vi "Evaluate Part 1.vi"() -> ()   [LabVIEW 2021]
uses:
  Proto/Module.lvclass
panel:
  out "Low Pulses":i32
  out "High Pulses":i32
  out "delimited string":string
  out "High x Low":u64
  in  "Input":string
  # "2532512431 too high"
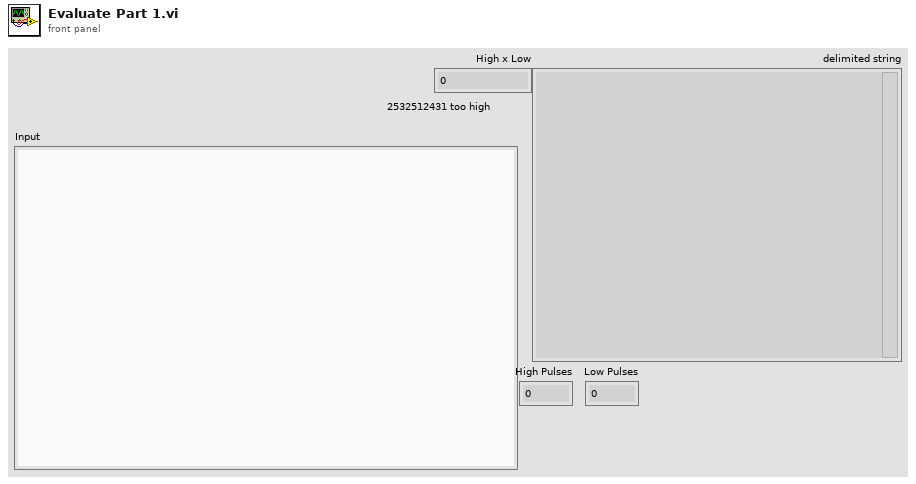
[diagram p1: front panel]
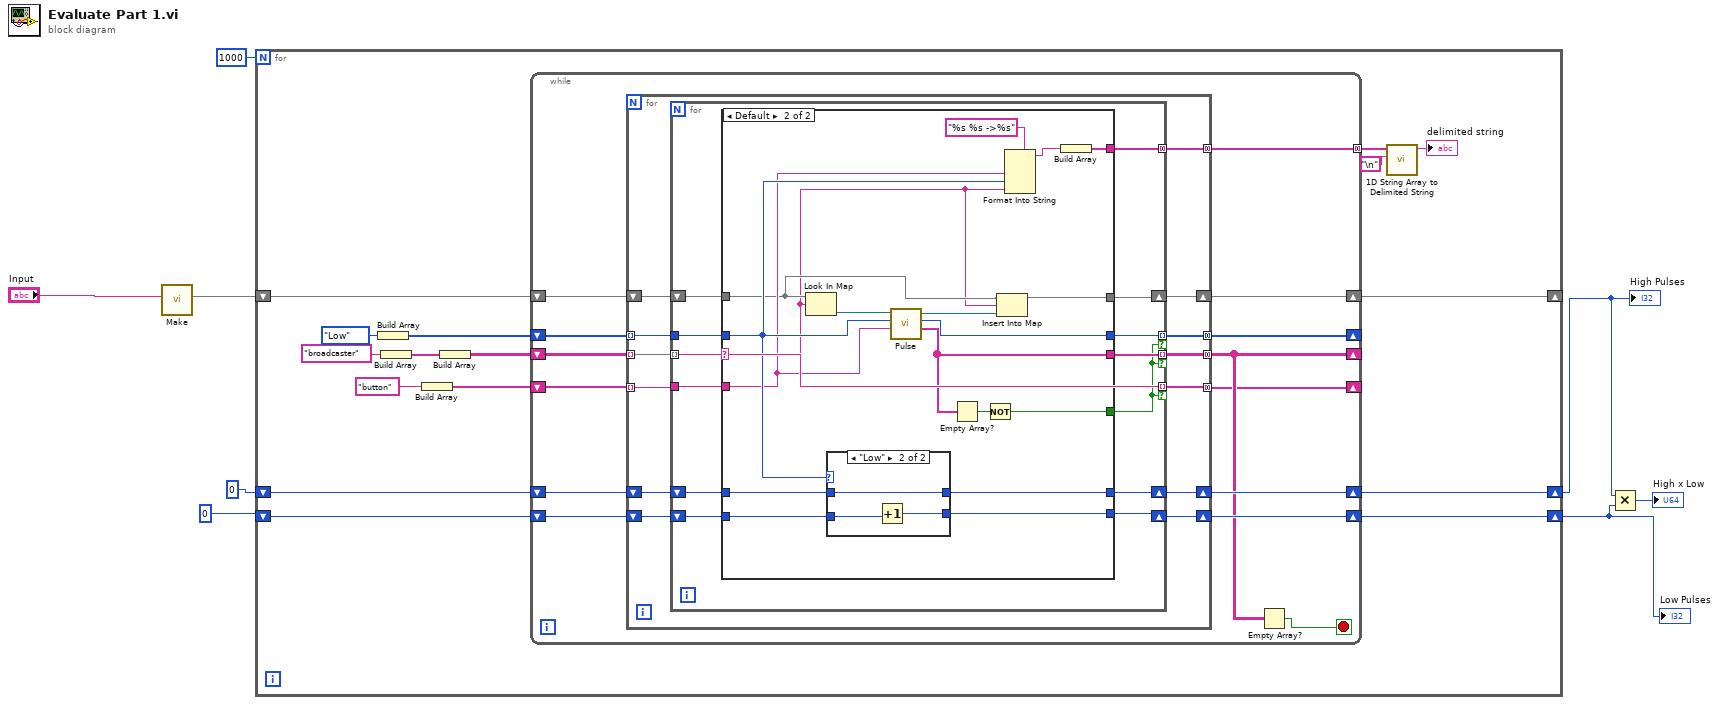
[diagram p0: block diagram]
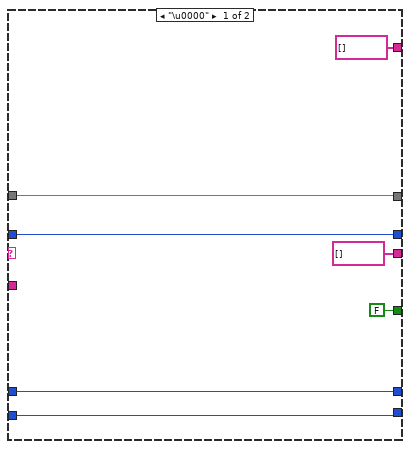
[diagram p2: hidden frame]
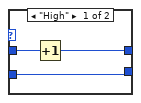
[diagram p3: hidden frame]
diagram:
  n1 = call "Make.vi"("Input"="Input") -> ("map"=w8:map{string, refnum<class "Module.lvclass">})  [unwired: 8 in, 2 out]
  n2 = for {
    N: 1000 -> [_]
    shift-right: [w11] -> _
    shift-left: w8 -> [w24]
    shift-right: [w18] -> w6
    shift-left: u64 0 -> [w10]
    shift-right: [w12] -> w4
    shift-left: u64 0 -> [w9]
    n3 = Build Array(enum16{"Low", "High"}."Low" ("Pulse In")) -> (w19:enum16{"Low", "High"}[])
    n4 = Build Array("broadcaster" ("key")) -> (w21:string[])
    n5 = Build Array("button" ("Sender")) -> (w14:string[])
    n6 = Build Array(w21) -> (w13:string[][])
    n7 = while {
      shift-right: [w29] -> _
      shift-left: w13 -> [w36]
      shift-right: [w34] -> _
      shift-left: w19 -> [w37]
      shift-right: [w32] -> w18
      shift-left: w10 -> [w33]
      shift-right: [w30] -> w12
      shift-left: w9 -> [w31]
      tunnel: [w28] -> w17 mode=concatenating
      shift-right: [w27] -> _
      shift-left: w14 -> [w35]
      shift-right: [w26] -> w11
      shift-left: w24 -> [w38]
      stop <- w25 stop-if-true
      n8 = for {
        tunnel: w36 -> [w51] mode=indexing
        tunnel: w37 -> [w49] mode=indexing
        tunnel: [w48] -> w29 mode=concatenating
        tunnel: [w46] -> w34 mode=concatenating
        shift-right: [w44] -> w32
        shift-left: w33 -> [w45]
        shift-right: [w42] -> w30
        shift-left: w31 -> [w43]
        tunnel: [w41] -> w28 mode=concatenating
        tunnel: w35 -> [w47] mode=indexing
        tunnel: [w40] -> w27 mode=concatenating
        shift-right: [w39] -> w26
        shift-left: w38 -> [w50]
        n9 = for {
          tunnel: w51 -> [w54] mode=indexing
          tunnel: [w53] -> w48 mode=indexing if=w52
          shift-right: [w62] -> w44
          shift-left: w45 -> [w63]
          shift-right: [w60] -> w42
          shift-left: w43 -> [w61]
          tunnel: [w57] -> w41 mode=concatenating
          tunnel: w47 -> [w58]
          tunnel: [w54] -> w40 mode=indexing if=w52
          shift-right: [w55] -> w39
          shift-left: w50 -> [w56]
          tunnel: w49 -> [w59]
          tunnel: [w64] -> w46 mode=indexing if=w52
          n10 = case shown="Default" w54 {
            selector: w54 -> [_ w77]
            tunnel: [w70 w88] -> w64
            tunnel: w63 -> [w67 w87]
            tunnel: [w67 w86] -> w62
            tunnel: w61 -> [w66 w85]
            tunnel: [w66 w84] -> w60
            tunnel: w59 -> [w70 w83]
            tunnel: w58 -> [_ w82]
            tunnel: [string[] [] w72] -> w57
            tunnel: w56 -> [w71 w79]
            tunnel: [w71 w78] -> w55
            tunnel: [string[] [] ("Receivers") w75] -> w53
            tunnel: [FALSE w73] -> w52
            frame "\u0000" {
            }
            frame Default {
              n11 = Look In Map(map=w79, key=w77) -> (value=w89:refnum<class "Module.lvclass">)  [unwired: 1 in, 1 out]
              n12 = case shown="\"Low\"" w83 {
                tunnel: w87 -> [w92 w95]
                tunnel: [w91 w95] -> w86
                tunnel: w85 -> [w90 w94]
                tunnel: [w90 w93] -> w84
                frame "High" {
                  n13 = Increment(x=w92) -> (x+1=w91:u64)
                }
                frame "Low" {
                  n14 = Increment(x=w94) -> (x+1=w93:u64)
                }
              }
              n15 = call-dynamic "Pulse.vi"("Sender"=w82, "Pulse In"=w83, "Module In"=w89) -> ("Receivers"=w75:string[], "Pulse Out"=w88:enum16{"Low", "High"}, "Module Out"=w76:refnum<class "Module.lvclass">)  [unwired: 5 in, 1 out]
              n16 = Empty Array?(array=w75) -> (empty?=w74:bool)
              n17 = Not(x=w74) -> (.not. x?=w73:bool)
              n18 = Insert Into Map(map in=w79, key=w77, value=w76) -> (map out=w78:map{string, refnum<class "Module.lvclass">})  [unwired: 2 out]
              n19 = Format Into String(format string="%s %s ->%s", w82, w83, w77) -> (resulting string=w81:string)  [unwired: 2 in, 1 out]
              n20 = Build Array(w81) -> (w72:string[])
            }
          }
        }
      }
      n21 = Empty Array?(array=w29) -> (empty?=w25:bool)
    }
    n22 = call <vilib>:"1D String Array to Delimited String.vi"("delimiter"="\n", "string array"=w17) -> ("delimited string"=→"delimited string":string)  [unwired: 9 in]
  }
  "High Pulses" <- w6
  "Low Pulses" <- w4
  n23 = Multiply(x=w6, y=w4) -> (x*y=→"High x Low":u64)
